vi "RTS Check Close TDMS File.vi"(8 "error in (no error)":errorcluster, 10 "CSV File Location In":path, 11 "Byte Stream In":refnum<file>) -> (0 "error out":errorcluster, 2 "CSV File Location Out":path, 3 "Byte Stream Out":refnum<file>)   [LabVIEW 2016]
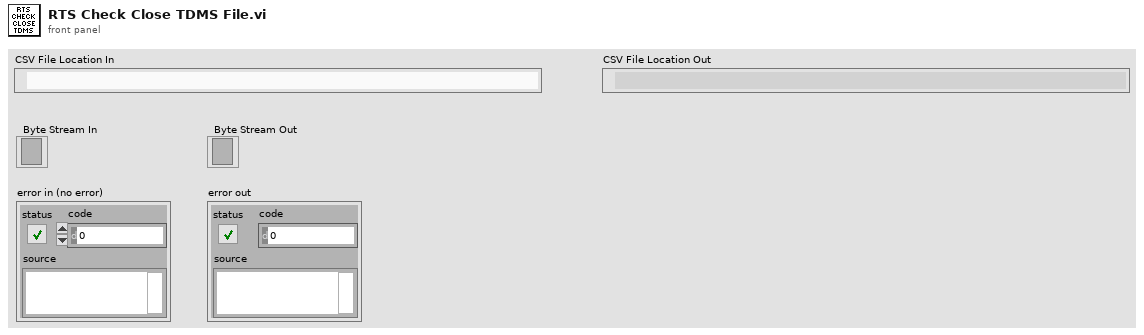
[diagram p1: front panel]
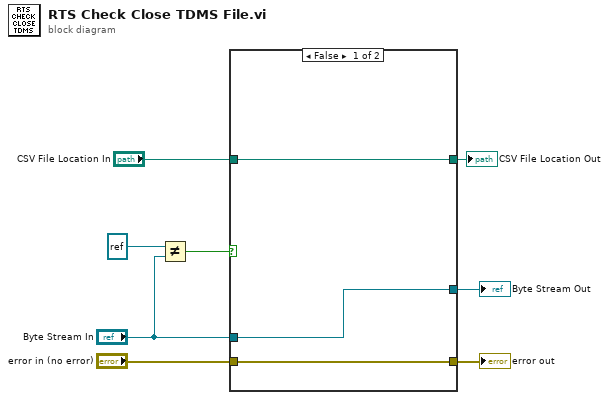
[diagram p0: block diagram]
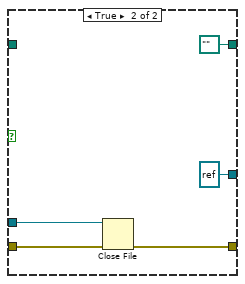
[diagram p2: hidden frame]
diagram:
  n1 = Not Equal?(x=refnum<file> refnum, y="Byte Stream In") -> (x != y?=w5:bool)
  n2 = case shown="False" w5 {
    tunnel: "error in (no error)" -> [w11 w16]
    tunnel: [w11 w15] -> w8
    tunnel: "Byte Stream In" -> [w10 w13]
    tunnel: [w10 refnum<file> refnum ("Byte Stream File in")] -> w3
    tunnel: "CSV File Location In" -> [w9 _]
    tunnel: [w9 path "" ("CSV File Location In")] -> w1
    frame False {
    }
    frame True {
      n3 = Close File(refnum=w13, error in=w16) -> (error out=w15:errorcluster)  [unwired: 1 out]
    }
  }
  "error out" <- w8
  "Byte Stream Out" <- w3
  "CSV File Location Out" <- w1
